vi "AdjustPIDParameters.vi"() -> ()   [LabVIEW 2018, in "JULABO DeviceDriver.lvlib"]
doc: "This example shows how to change control parameters in the unit"
uses:
  JULABO DeviceDriver.lvlib
panel:
  out "error out":errorcluster caption="Fehler (Ausgang)"
  in  "Adjust":bool
  in  "Tv (0s)":u16 max=999
  in  "Tn (3s)":u16=3 min=3 max=9999
  in  "Xp (0.6K)":dbl=0.6 min=0.1 max=99.9
  out "Selftuning (out)":enum16{"OFF", "ONCE", "ALWAYS"}(ring)
  out "InternalTv (out)":u16
  out "InternalTn (out)":u16
  out "InternalXp (out)":dbl
  in  "VISA resource name":refnum<visa-resource-name>="COM3"
  in  "Reset / Default (T: Both)":bool=TRUE
  in  "ID Query? (T: Yes)":bool=TRUE
  in  "RS485-Address (128: RS232)":u32=128
  in  "Serial Configuration":T1={"Baud Rate"=4800, "Parity"=2, "Data Bits"=7, "Stop Bits"=10, "Flow Control"=2} {"Flow Control" items=["None", "XON/XOFF", "RTS/CTS", "XON/XOFF & RTS/CTS", "DTR/DSR", "XON/XOFF & DTR/DSR"]; "Stop Bits" items=["1.0"=10, "1.5"=15, "2.0"=20]; "Data Bits" items=["7"=7, "8"=8]; "Parity" items=["None", "Odd", "Even", "Mark", "Space"]; "Baud Rate" items=["300"=300, "600"=600, "1200"=1200, "2400"=2400, "4800"=4800, "9600"=9600, "19200"=19200]}
  in  "Stop":bool
  in  "Read cycle (ms)":u32=1000
  # "1. Select the COM-Port and adjust the serial\nconfiguration for your instrument\n2. Adjust the Read cycle\n3. Start the VI by pressing the \"Start\" -Button\n( Arrow button on the top-left corner)\n4. To stop the execution press the \"Stop\" button"
  # "Adjust parameters"
  # "Read parameters"
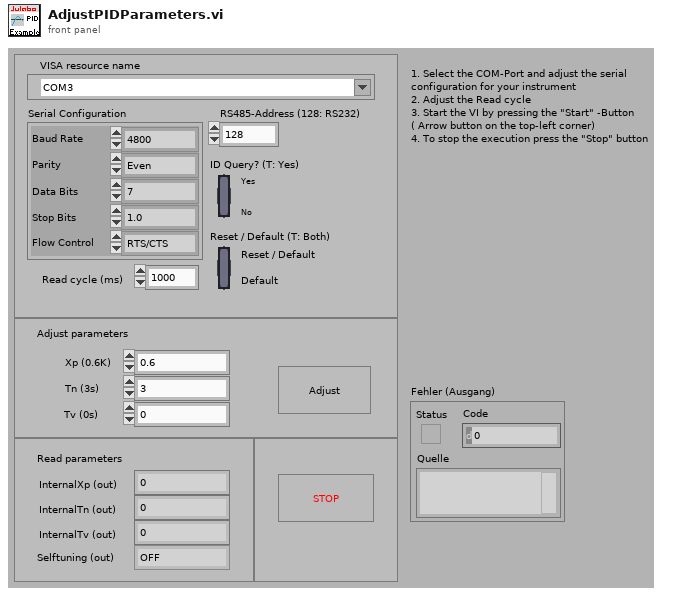
[diagram p1: front panel]
types:
  T1 = cluster{"Baud Rate":u32, "Parity":u16, "Data Bits":u16, "Stop Bits":u16, "Flow Control":u16}
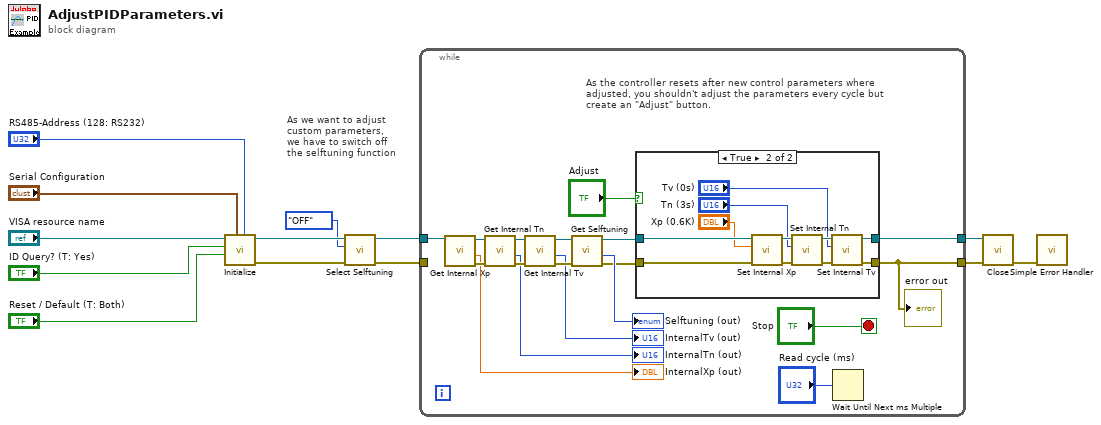
[diagram p0: block diagram]
diagram:
  # "As we want to adjust\ncustom parameters,\nwe have to switch off\nthe selftuning function"
  n1 = call "Initialize.vi"("RS485-Address (128: RS232)"="RS485-Address (128: RS232)", "Serial Configuration"="Serial Configuration", "Reset / Default (T: Both)"="Reset / Default (T: Both)", "ID Query? (T: Yes)"="ID Query? (T: Yes)", "VISA resource name"="VISA resource name") -> ("error out"=w4:errorcluster, "VISA resource name out"=w5:refnum<visa-resource-name>)  [unwired: 5 in]
  n2 = call "Select Selftuning.vi"("error in (no error)"=w4, "Selftuning (0: OFF)"=enum16{"OFF", "ONCE", "ALWAYS"}."OFF", "VISA resource name"=w5) -> ("error out"=w3:errorcluster, "VISA resource name out"=w2:refnum<visa-resource-name>)  [unwired: 7 in]
  n3 = while {
    tunnel: w2 -> [w19]
    tunnel: [w15] -> w13
    tunnel: [w14] -> w12
    tunnel: w3 -> [_]
    stop <- "Stop" stop-if-true
    # "As the controller resets after new control parameters where\nadjusted, you shouldn't adjust the parameters every cycle but\ncreate an \"Adjust\" button."
    n4 = call "Get Internal Xp.vi"("VISA resource name in"=w19) -> ("error out"=w28:errorcluster, "InternalXp (out)"=→"InternalXp (out)":dbl, "VISA resource name out"=w29:refnum<visa-resource-name>)  [unwired: 8 in]
    n5 = call "Get Internal Tn.vi"("error in"=w28, "VISA resource name in"=w29) -> ("error out"=w26:errorcluster, "InternalTn (out)"=→"InternalTn (out)":u16, "VISA resource name out"=w27:refnum<visa-resource-name>)  [unwired: 7 in]
    n6 = call "Get Internal Tv.vi"("error in"=w26, "VISA resource name in"=w27) -> ("error out"=w24:errorcluster, "InternalTv (out)"=→"InternalTv (out)":u16, "VISA resource name out"=w25:refnum<visa-resource-name>)  [unwired: 7 in]
    n7 = call "Get Selftuning.vi"("error in"=w24, "VISA resource name in"=w25) -> ("error out"=w17:errorcluster, "Selftuning (out)"=→"Selftuning (out)":enum16{"OFF", "ONCE", "ALWAYS"}, "VISA resource name out"=w18:refnum<visa-resource-name>)  [unwired: 7 in]
    n8 = case shown="True" "Adjust" {
      tunnel: w18 -> [w33 w40]
      tunnel: w17 -> [w32 w39]
      tunnel: [w33 w38] -> w15
      tunnel: [w32 w37] -> w14
      frame False {
      }
      frame True {
        n9 = call "Set Internal Xp.vi"("error in (no error)"=w39, "Xp (0.6K)"="Xp (0.6K)", "VISA resource name"=w40) -> ("error out"=w42:errorcluster, "VISA resource name out"=w41:refnum<visa-resource-name>)  [unwired: 7 in]
        n10 = call "Set Internal Tn.vi"("error in (no error)"=w42, "Tn (3s)"="Tn (3s)", "VISA resource name"=w41) -> ("error out"=w44:errorcluster, "VISA resource name out"=w43:refnum<visa-resource-name>)  [unwired: 7 in]
        n11 = call "Set Internal Tv.vi"("error in (no error)"=w44, "Tv (0s)"="Tv (0s)", "VISA resource name"=w43) -> ("error out"=w37:errorcluster, "VISA resource name out"=w38:refnum<visa-resource-name>)  [unwired: 7 in]
      }
    }
    "error out" <- w14
    n12 = Wait Until Next ms Multiple(millisecond multiple="Read cycle (ms)") -> ()  [unwired: 1 out]
  }
  n13 = call "Close.vi"("error in (no error)"=w12, "VISA resource name"=w13) -> ("error out"=w9:errorcluster)  [unwired: 9 in]
  n14 = call <vilib>:"Simple Error Handler.vi"("error in (no error)"=w9) -> ()  [unwired: 4 in, 5 out]
